vi "Initialise.vi"(6 "ProjectPath":path, 8 "error in (no error)":errorcluster, 11 "Interface Name":string) -> (0 "error out":errorcluster, 3 "Class Out":refnum<class "CreateClass.lvclass">)   [LabVIEW 2020, in "Mermaid.lvlib" / "CreateClass.lvclass"]
uses:
  CreateClass.lvclass
  CreateClass.lvclass/CreateClass.ctl
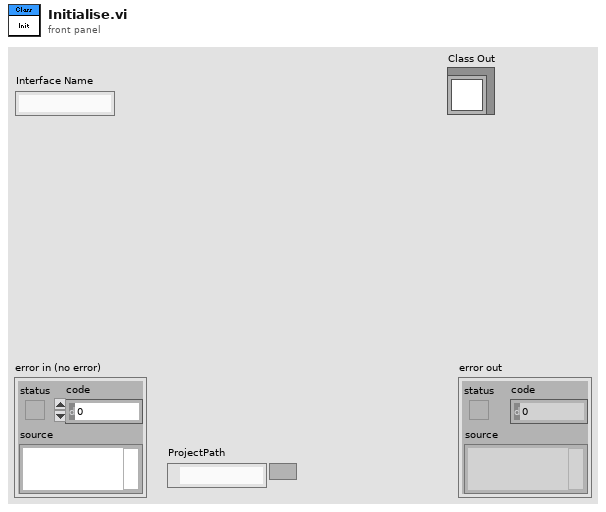
[diagram p1: front panel]
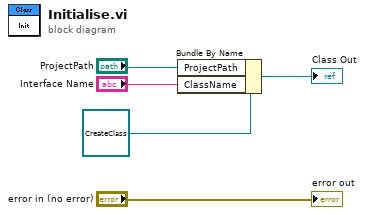
[diagram p0: block diagram]
diagram:
  n1 = Bundle By Name(cluster=refnum<class "CreateClass.lvclass"> refnum ("CreateClass.lvclass"), "ProjectPath"="ProjectPath", "ClassName"="Interface Name") -> (→"Class Out":refnum<class "CreateClass.lvclass">)
  "error out" <- "error in (no error)"
